vi "XiXi-1(Add DBL[]).vi"(10 "X[-1]":dbl[](array[numeric]), 11 "Xi":dbl[][](array[numeric])) -> (3 "Yi":dbl[][](array[numeric]) format="%.2f")   [LabVIEW 2012]
doc: "Calculate sums of consecutive array elements. 0th element of output is equal to x(0)+ x(-1), where x(-1) is an optional scalar input that defaults to zero."
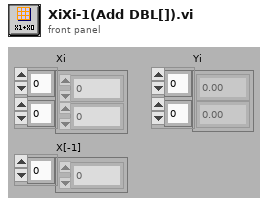
[diagram p1: front panel]
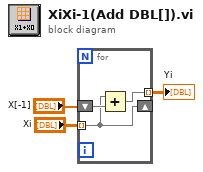
[diagram p0: block diagram]
diagram:
  n1 = for {
    shift-right: [w5] -> _
    shift-left: "X[-1]" -> [w6]
    tunnel: "Xi" -> [w5] mode=indexing
    tunnel: [w4] -> w1 mode=indexing
    n2 = Add(x=w5, y=w6) -> (x+y=w4:dbl[])
  }
  "Yi" <- w1
